vi "Stim.vi"(11 "Tstim ON":dbl) -> (3 "Vstim":cluster{"Test":dbl[], "Train":dbl[], "#s":dbl})   [LabVIEW 2016]
uses:
  <vilib>/measure/NI_MABase.lvlib
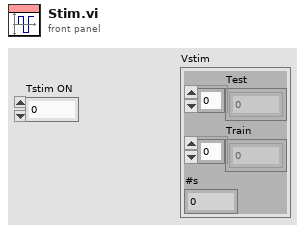
[diagram p1: front panel]
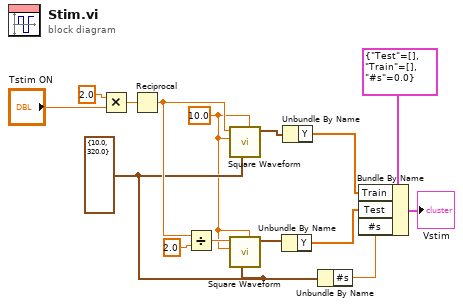
[diagram p0: block diagram]
diagram:
  w5 = cluster{"Fs":dbl, "#s":dbl} {"Fs"=10.0, "#s"=320.0} ("sampling info")
  w1 = 10.0 ("amplitude")
  n1 = Multiply(x=2.0, y="Tstim ON") -> (x*y=w8:dbl)
  n2 = Reciprocal(x=w8) -> (1/x=w10:dbl)
  n3 = Divide(x=w10, y=2.0) -> (x/y=w11:dbl)
  n4 = call <vilib>:"Square Waveform.vi"("offset"=w1, "sampling info"=w5, "amplitude"=w1, "frequency"=w10) -> ("signal out"=w14:waveform(dbl))  [unwired: 6 in, 1 out]
  n5 = call <vilib>:"Square Waveform.vi"("offset"=w1, "sampling info"=w5, "amplitude"=w1, "frequency"=w11) -> ("signal out"=w13:waveform(dbl))  [unwired: 6 in, 1 out]
  n6 = Unbundle By Name(w13) -> ("Y"=w2:dbl[])
  n7 = Unbundle By Name(w14) -> ("Y"=w3:dbl[])
  n8 = Unbundle By Name(w5) -> ("#s"=w6:dbl)
  n9 = Bundle By Name(cluster=cluster{"Test":dbl[], "Train":dbl[], "#s":dbl} {"Test"=[], "Train"=[], "#s"=0.0} ("input cluster"), "Train"=w3, "Test"=w2, "#s"=w6) -> (→"Vstim":cluster{"Test":dbl[], "Train":dbl[], "#s":dbl})
